vi "destroy.vi"(8 "error in (no error)":errorcluster, 11 "TaskController in":refnum<class "TaskController.lvclass">) -> (0 "error out":errorcluster, 2 "taskError":errorcluster, 3 "taskResult":refnum<class "ITask.lvclass">)   [LabVIEW 2023, in "TLC_Daemon.lvlib" / "TaskController.lvclass"]
doc: "Destroys the TaskController and returns the task outputs: Task out and Error out.\n\nIf the task is running, this method forces it to stop. If the Destroy method is called before the task has been launched, or if the task fails to stop, the Task object originally provided to the New method is returned.\n\nSet 'destroyStopMechanism' to True to also trigger the destruction of the StopMechanism."
uses:
  TaskController.lvclass
  ITask/ITask.lvclass
  TaskController.lvclass/TaskController.ctl
  ITaskChannel/ITaskChannel.lvclass
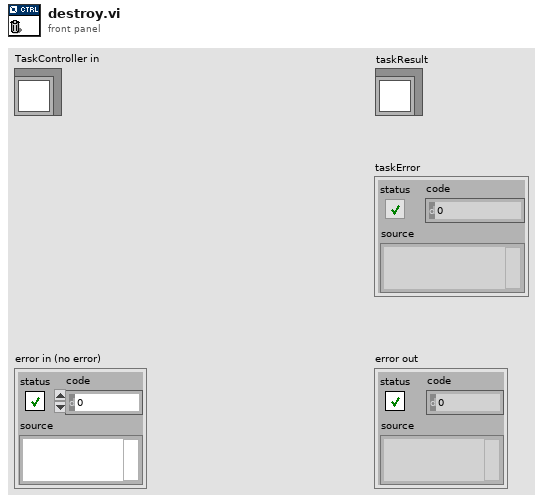
[diagram p1: front panel]
types:
  T1 = typedef "TLC_Daemon.lvlib/TaskController.lvclass/status.ctl" = enum16{"NotReady", "Ready", "Running", "Stopped", "Unknown"}
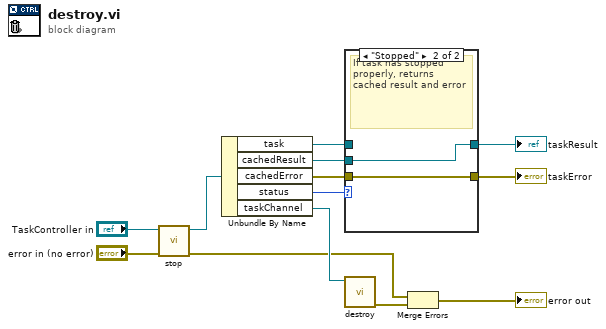
[diagram p0: block diagram]
diagram:
  n1 = call "stop.vi"("error in (no error)"="error in (no error)", "TaskController in"="TaskController in") -> ("error out"=w7:errorcluster, "TaskController out"=w12:refnum<class "TaskController.lvclass">)  [unwired: 8 in]
  n2 = Unbundle By Name(w12) -> ("task"=w1:refnum<class "ITask.lvclass">, "cachedResult"=w5:refnum<class "ITask.lvclass">, "cachedError"=w3:errorcluster, "status"=w6:T1, "taskChannel"=w11:refnum<class "ITaskChannel.lvclass">)
  n3 = case shown="\"Stopped\"" w6 {
    tunnel: w5 -> [_ w16]
    tunnel: [w14 w16] -> w4
    tunnel: w3 -> [_ w15]
    tunnel: [_ w15] -> w2
    tunnel: w1 -> [w14 _]
    frame Default {
    }
    frame "Stopped" {
      # "If task has stopped properly, returns cached result and error"
    }
  }
  "taskResult" <- w4
  "taskError" <- w2
  n4 = call-dynamic "destroy.vi"("ITaskStopMechanism in"=w11) -> ("error out"=w10:errorcluster)  [unwired: 9 in, 1 out]
  n5 = Merge Errors(w7, w10) -> (→"error out":errorcluster)
